vi "Convert to GUID.vi"(11 "Key":string) -> (3 "GUID":string)   [LabVIEW 2018]
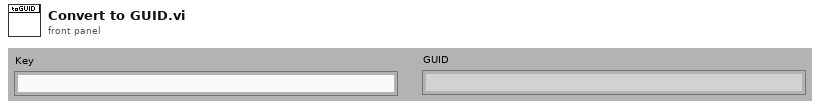
[diagram p1: front panel]
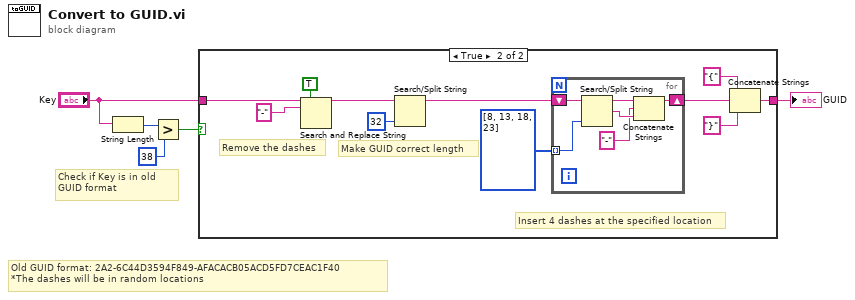
[diagram p0: block diagram]
diagram:
  # "Old GUID format: 2A2-6C44D3594F849-AFACACB05ACD5FD7CEAC1F40\n*The dashes will be in random locations"
  # "Check if Key is in old GUID format"
  n1 = String Length(string="Key") -> (length=w3:i32)
  n2 = Greater?(x=w3, y=38) -> (0:w1:bool)
  n3 = case shown="True" w1 {
    tunnel: [w6 w8] -> w5
    tunnel: "Key" -> [w6 w7]
    frame False {
    }
    frame True {
      # "Insert 4 dashes at the specified location"
      # "Make GUID correct length"
      # "Remove the dashes"
      n4 = Search and Replace String(replace all?=TRUE ("replace all? (F)"), input string=w7, search string="-") -> (result string=w15:string)  [unwired: 5 in, 3 out]
      n5 = Search/Split String(string=w15, offset (0)=32) -> (substring before match=w13:string)  [unwired: 1 in, 2 out]
      n6 = for {
        shift-right: [w22] -> w9
        shift-left: w13 -> [w23]
        tunnel: i32[] [8, 13, 18, 23] -> [w18] mode=indexing
        n7 = Search/Split String(string=w23, offset (0)=w18) -> (substring before match=w21:string, match + rest of string=w20:string)  [unwired: 1 in, 1 out]
        n8 = Concatenate Strings(w21, "-" ("string"), w20) -> (w22:string)
      }
      n9 = Concatenate Strings("{" ("string"), w9, "}" ("string")) -> (w8:string)
    }
  }
  "GUID" <- w5
